vi "Init.vi"(8 "error in (no error)":errorcluster, 10 "index":i32, 11 "BC_Steady_2D_VIRef":refnum<class "NI_BC_Steady_2D_VIRef.lvclass">) -> (0 "error out":errorcluster, 3 "initialized BC_Steady_2D_VIRef":refnum<class "NI_BC_Steady_2D_VIRef.lvclass">)   [LabVIEW 2020, in "NI_PDE.lvlib" / "NI_BC_Steady_2D_VIRef.lvclass"]
uses:
  <vilib>/gmath/pde.llb/BCClass/BC_Steady_2D_VIRef/NI_BC_Steady_2D_VIRef.lvclass
  <vilib>/gmath/pde.llb/BCClass/Class Type.ctl
  <vilib>/gmath/pde.llb/Common/PDE_BC Type.ctl
  <vilib>/gmath/pde.llb/BCClass/BC_Steady_2D_VIRef/NI_BC_Steady_2D_VIRef.lvclass/NI_BC_Steady_2D_VIRef.ctl
  <vilib>/gmath/pde.llb/BCClass/NI_BC.lvclass
  <vilib>/gmath/NI_PDE.lvlib
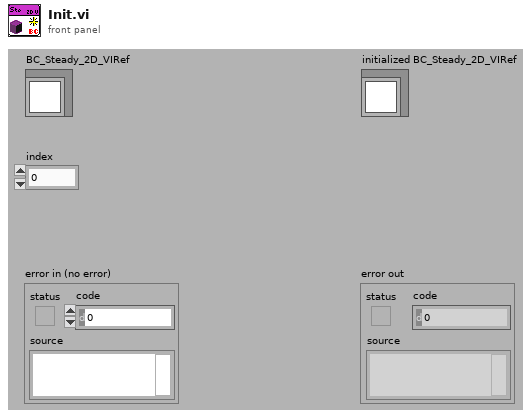
[diagram p1: front panel]
types:
  T1 = typedef "NI_PDE.lvlib/PDE_BC Type.ctl" = i32
  T2 = typedef "NI_PDE.lvlib/NI_BC.lvclass/Class Type.ctl" = i32
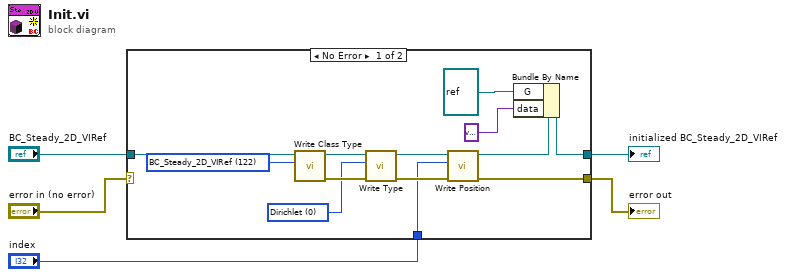
[diagram p0: block diagram]
diagram:
  n1 = case shown="No Error" "error in (no error)" {
    selector: "error in (no error)" -> [_ w19]
    tunnel: [w9 w20] -> w5
    tunnel: [w8 w19] -> w4
    tunnel: "BC_Steady_2D_VIRef" -> [w12 w20]
    tunnel: "index" -> [w11 _]
    frame No Error {
      w13 = T1 0 items=["Dirichlet", "Neumann"] ("BC type")
      w14 = T2 122 items=["BC"=0, "BC_Steady"=100, "BC_Steady_2D"=120, "BC_Steady_2D_Numeric"=121, "BC_Steady_2D_VIRef"=122, "BC_Evolut"=200, "BC_Evolut_1D"=210, "BC_Evolut_1D_Numeric"=211, "BC_Evolut_1D_VIRef"=212, "BC_Evolut_2D"=220, "BC_Evolut_2D_Numeric"=221, "BC_Evolut_2D_VIRef"=222] ("BC class type")
      n2 = call-dynamic "Write Class Type.vi"("BC class type"=w14, "BC.lvclass in"=w12) -> ("error out"=w15:errorcluster, "BC.lvclass out"=w18:refnum<class "NI_BC_Steady_2D_VIRef.lvclass">)  [unwired: 1 in, 7 out]
      n3 = call-dynamic "Write Type.vi"("error in (no error)"=w15, "BC type"=w13, "BC.lvclass in"=w18) -> ("error out"=w16:errorcluster, "BC.lvclass out"=w17:refnum<class "NI_BC_Steady_2D_VIRef.lvclass">)  [unwired: 7 out]
      n4 = call-dynamic "Write Position.vi"("error in (no error)"=w16, "BC position 2D"=w11, "BC_Steady_2D.lvclass in"=w17) -> ("error out"=w8:errorcluster, "BC_Steady_2D.lvclass out"=w10:refnum<class "NI_BC_Steady_2D_VIRef.lvclass">)  [unwired: 7 out]
      n5 = Bundle By Name(cluster=w10, "G"=refnum<vi> refnum, "data"=variant) -> (w9:refnum<class "NI_BC_Steady_2D_VIRef.lvclass">)
    }
    frame Error {
    }
  }
  "initialized BC_Steady_2D_VIRef" <- w5
  "error out" <- w4
